vi "CalcCoordinates.vi"(9 "SwerveAngles":dbl, 10 "Y":dbl, 11 "X":dbl) -> (2 "Y'":dbl, 3 "X'":dbl)   [LabVIEW 2017]
uses:
  AutoGlobals.vi
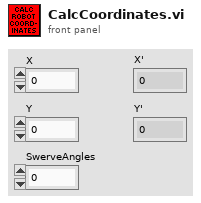
[diagram p1: front panel]
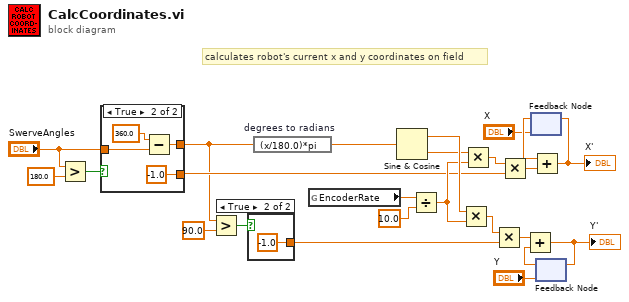
[diagram p0: block diagram]
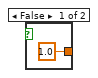
[diagram p2: hidden frame]
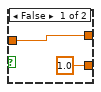
[diagram p3: hidden frame]
diagram:
  # "calculates robot's current x and y coordinates on field"
  n1 = Greater?(x="SwerveAngles", y=180.0) -> (0:w20:bool)
  n2 = case shown="True" w20 {
    tunnel: "SwerveAngles" -> [w26 w28]
    tunnel: [w26 w30] -> w4
    tunnel: [1.0 -1.0] -> w6
    frame False {
    }
    frame True {
      n3 = Subtract(x=360.0, y=w28) -> (x-y=w30:dbl)
    }
  }
  n4 = Greater?(x=w4, y=90.0) -> (0:w17:bool)
  n5 = case shown="True" w17 {
    tunnel: [1.0 -1.0] -> w3
    frame False {
    }
    frame True {
    }
  }
  n6 = expression code="(x/180.0)*pi" "degrees to radians"(w4) -> (w24:dbl)
  n7 = global read "AutoGlobals.vi" "EncoderRate"() -> (w8:dbl)
  n8 = Sine & Cosine(0:w24) -> (1:w23:dbl, 2:w21:dbl)
  n9 = Divide(x=w8, y=10.0) -> (x/y=w7:dbl)
  n10 = Multiply(x=w23, y=w7) -> (x*y=w22:dbl)
  n11 = Multiply(x=w21, y=w7) -> (x*y=w16:dbl)
  n12 = Multiply(x=w22, y=w3) -> (x*y=w15:dbl)
  n13 = Multiply(x=w16, y=w6) -> (x*y=w13:dbl)
  n14 = feedback #1("X") -> (w12:dbl)
  n15 = Add(x=w12, y=w13) -> (x+y=w2:dbl)
  "X'" <- w2
  n16 = feedback-in #1(w2) -> ()
  n17 = feedback #2("Y") -> (w14:dbl)
  n18 = Add(x=w15, y=w14) -> (x+y=w1:dbl)
  "Y'" <- w1
  n19 = feedback-in #2(w1) -> ()
